vi "Read Assertion Type.vi"(11 "Test Assertion Result In":refnum<class "Assertion Result.lvclass">) -> (2 "Assertion Type":T1, 3 "Test Assertion Result Out":refnum<class "Assertion Result.lvclass">)   [LabVIEW 2020, in "Assertion Result.lvclass"]
uses:
  Assertion Result.lvclass
  TypeDefs/Assertion Type.ctl
  Assertion Result.lvclass/Assertion Result.ctl
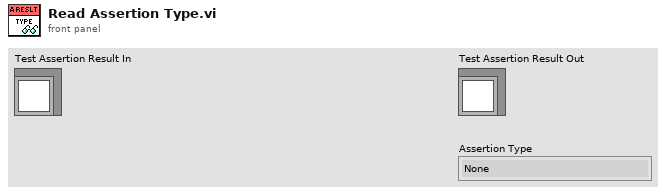
[diagram p1: front panel]
types:
  T1 = typedef "Assertion Result.lvclass/Assertion Type.ctl" = enum16{"None", "Pass", "Fail", "Skip", "Pass if Equal", "Fail if Equal", "Pass if Error", "Fail if Error", "Pass if", "Fail if"}
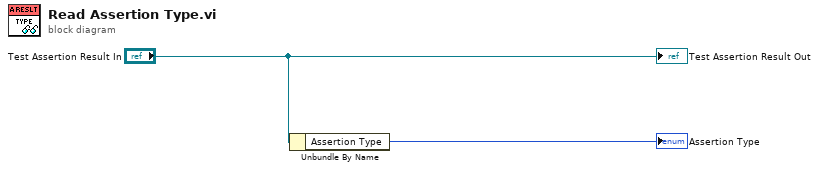
[diagram p0: block diagram]
diagram:
  n1 = Unbundle By Name("Test Assertion Result In") -> ("Assertion Type"=→"Assertion Type":T1)
  "Test Assertion Result Out" <- "Test Assertion Result In"
